vi "disclaimer.vi"() -> ()   [LabVIEW 2020]
panel:
  in  "acknoledge Button":bool
  out "String":string
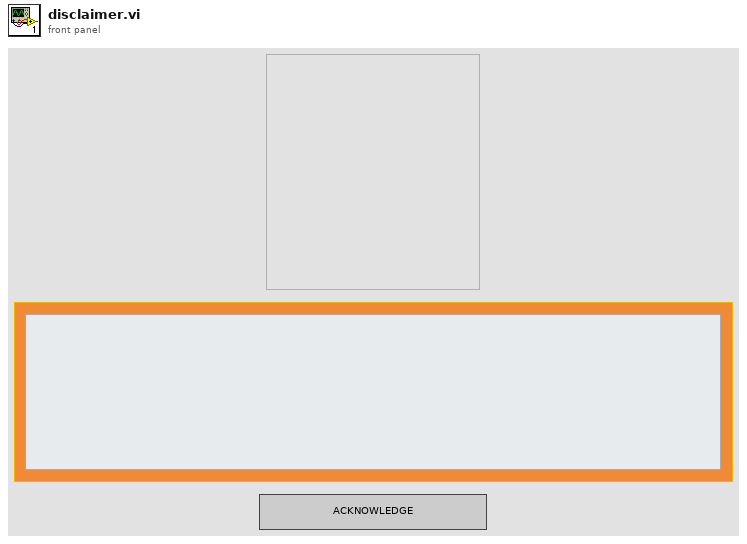
[diagram p1: front panel]
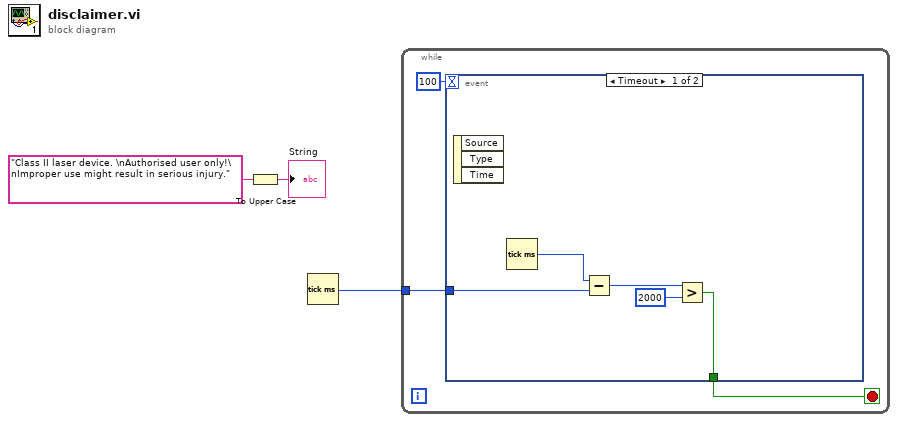
[diagram p0: block diagram]
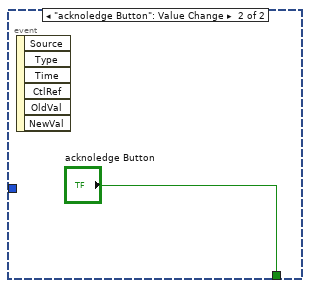
[diagram p2: hidden frame]
diagram:
  n1 = To Upper Case(1:"Class II laser device. \nAuthorised user only!\nImproper use might result in serious injury." ("String")) -> (0:→"String":string)
  n2 = Tick Count (ms)() -> (millisecond timer value=w1:u32)
  n3 = while {
    tunnel: w1 -> [w4]
    stop <- w6 stop-if-true
    n4 = event shown="[0] Timeout" {
      selector: _ -> [_ _]
      dyn-events: _ -> [_ _]
      timeout: 100 -> [_ _]
      tunnel: [w7 "acknoledge Button"] -> w6
      tunnel: w4 -> [w10 _]
      event Timeout {
        n5 = event-data() -> ()  [unwired: 1 in, 3 out]
        n6 = Tick Count (ms)() -> (millisecond timer value=w11:u32)
        n7 = Subtract(x=w11, y=w10) -> (x-y=w9:u32)
        n8 = Greater?(x=w9, y=u32 2000) -> (0:w7:bool)
      }
      event "acknoledge Button": Value Change {
        n9 = event-data() -> ()  [unwired: 1 in, 6 out]
      }
    }
  }
